vi "SUB_WR_Telnet.vi"(4 "Find this String":string, 5 "data in":string, 6 "timeout ms":i32=25000, 7 "telnet connection":T1) -> (1 "Found":bool, 2 "msg out":string, 3 "telnet connection out":T1)   [LabVIEW 2011]
uses:
  <vilib>/addons/internet/telnet/telnet.llb/Telnet Session.ctl
  <vilib>/addons/internet/NI_InternetTK_Core_VIs.lvlib
panel:
  out "error out":errorcluster
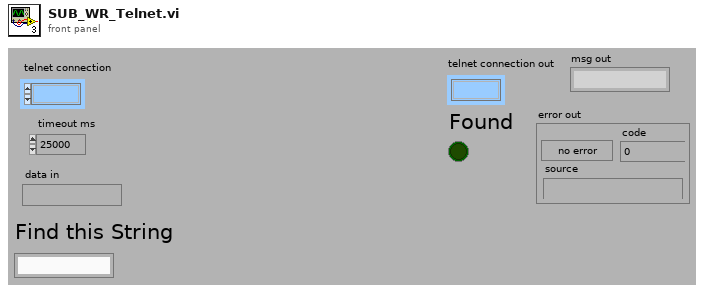
[diagram p1: front panel]
types:
  T1 = typedef "Telnet Session.ctl" = refnum<k1>
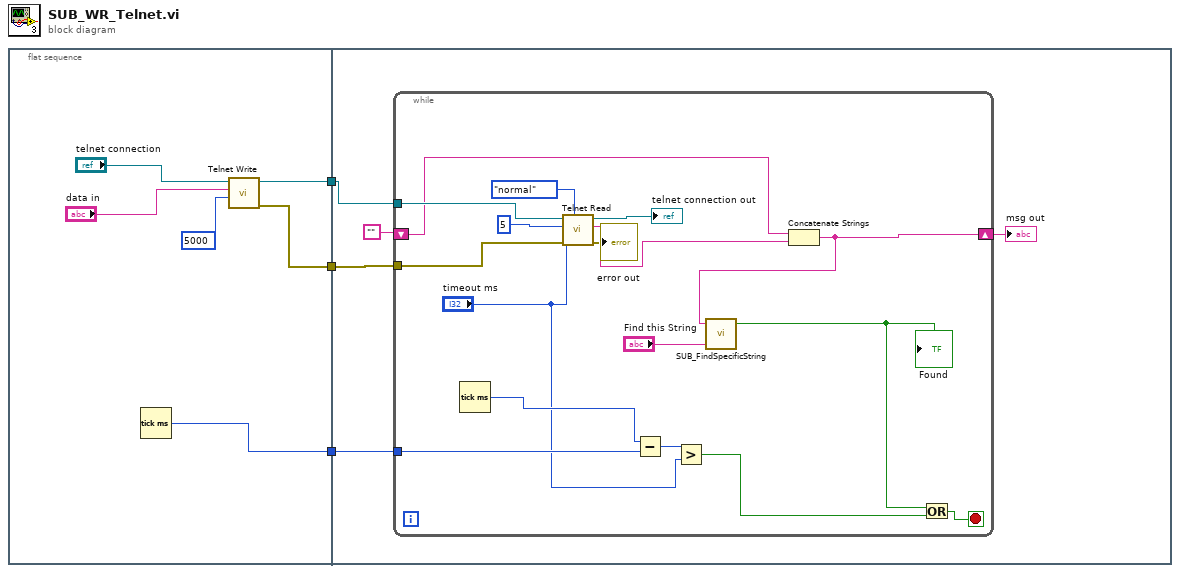
[diagram p0: block diagram]
diagram:
  n1 = flat-sequence {
    tunnel: [w7] -> w3
    tunnel: [w6] -> w2
    tunnel: [w5] -> w1
    tunnel: w3 -> [w14]
    tunnel: w2 -> [w13]
    tunnel: w1 -> [w11]
    frame #0 {
      n2 = Tick Count (ms)() -> (millisecond timer value=w5:u32)
      n3 = call <vilib>:"Telnet Write.vi"("timeout ms (25000)"=5000, "data in"="data in", "telnet connection"="telnet connection") -> ("error out"=w6:errorcluster, "telnet connection out"=w7:T1)  [unwired: 4 in, 1 out]
    }
    frame #1 {
      n4 = while {
        tunnel: w14 -> [w28]
        tunnel: w13 -> [w27]
        shift-right: [w23] -> w10
        shift-left: "" -> [w24]
        tunnel: w11 -> [w21]
        stop <- w18 stop-if-true
        n5 = Tick Count (ms)() -> (millisecond timer value=w22:u32)
        n6 = call <vilib>:"Telnet Read.vi"("read mode (normal)"=enum16{"normal", "line", "buffered"}."normal", "error in (no error)"=w27, "timeout ms (25000)"="timeout ms", "bytes to read"=5, "telnet connection"=w28) -> ("error out"=→"error out":errorcluster, "data out"=w25:string, "telnet connection out"=→"telnet connection out":T1)  [unwired: 2 in]
        n7 = Subtract(x=w22, y=w21) -> (x-y=w20:u32)
        n8 = Greater?(x=w20, y="timeout ms") -> (0:w16:bool)
        n9 = Concatenate Strings(w24, w25) -> (w23:string)
        n10 = call "SUB_FindSpecificString.vi"("Find this String"="Find this String", "String data"=w23) -> ("Found"=w17:bool)  [unwired: 2 in, 1 out]
        "Found" <- w17
        n11 = Or(x=w17, y=w16) -> (x .or. y?=w18:bool)
      }
      "msg out" <- w10
    }
  }
